vi "Update Command Data.vi"(8 "error in (no error)":errorcluster, 11 "Async RT-RT Message in":refnum<class "Async RT-RT Message.lvclass">) -> (0 "error out":errorcluster, 3 "Async RT-RT Message out":refnum<class "Async RT-RT Message.lvclass">)   [LabVIEW 2020, in "BCI-1553 API.lvlib" / "Async RT-RT Message.lvclass"]
uses:
  Async RT-RT Message.lvclass
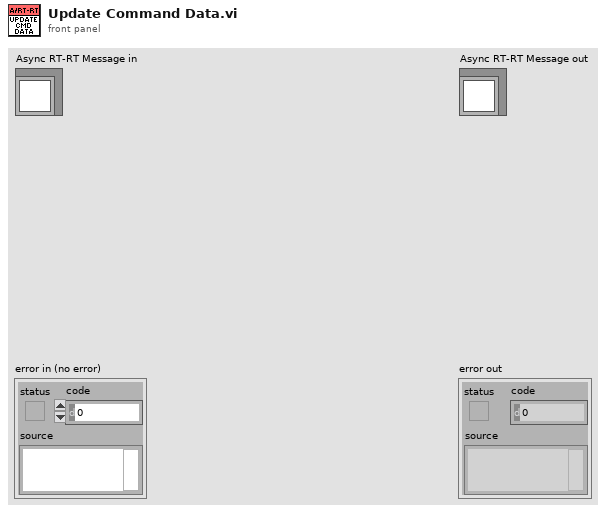
[diagram p1: front panel]
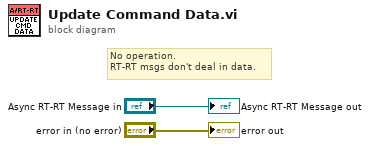
[diagram p0: block diagram]
diagram:
  # "No operation.\nRT-RT msgs don't deal in data."
  "error out" <- "error in (no error)"
  "Async RT-RT Message out" <- "Async RT-RT Message in"
